vi "LCC Read Actual Value Unscaled.vi"(8 "error in (no error)":errorcluster caption="Fehler (Eingang, kein Fehler)", 11 "Channel Handle":i64) -> (0 "error out":errorcluster caption="Fehler (Ausgang)", 3 "Actual Value Unscaled":dbl)   [LabVIEW 2021, in "labbCAN_Controller_API.lvlib"]
doc: "LCC_Func long LCC_CALL LCC_ReadActualValueUnscaled(dev_hdl ChanHdl, double *pfActualValueRaw);"
uses:
  labbCAN_Controller_API.lvlib
  labbCAN_Controller_API.dll
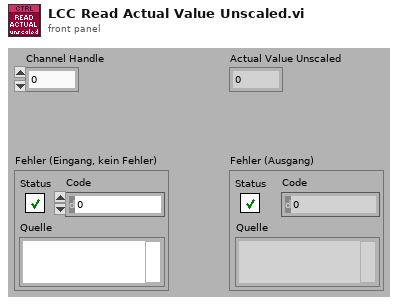
[diagram p1: front panel]
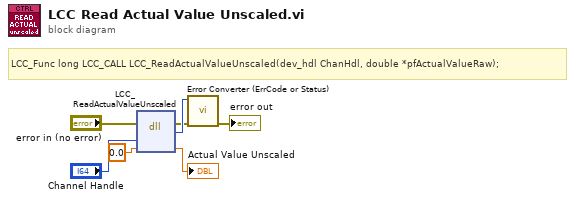
[diagram p0: block diagram]
diagram:
  # "LCC_Func long LCC_CALL LCC_ReadActualValueUnscaled(dev_hdl ChanHdl, double *pfActualValueRaw);"
  n1 = dll-call lib="C:/Users/olaja/AppData/Local/CETONI_SDK/labbCAN_Controller_API.*" fn="LCC_ReadActualValueUnscaled"(error in="error in (no error)", "ChanHdl"="Channel Handle", "pfActualValueRaw"=0.0) -> (error out=w2:errorcluster, "Rückgabetyp"=w3:i32, "pfActualValueRaw"=→"Actual Value Unscaled":dbl)  [unwired: 3 in, 1 out]
  n2 = call "Error Converter (ErrCode or Status).vi"("error in (no error)"=w2, "error code"=w3) -> ("error out"=→"error out":errorcluster)  [unwired: 9 in]
